vi "Write OCP Enable.vi"(8 "error in":errorcluster, 10 "OCP Enable":bool, 11 "Electronic Load in":refnum<class "Electronic Load.lvclass">) -> (0 "error out":errorcluster, 3 "Electronic Load out":refnum<class "Electronic Load.lvclass">)   [LabVIEW 2019, in "Electronic Load.lvlib" / "Electronic Load.lvclass"]
uses:
  Library/Electronic Load.lvclass
  C:/Users/Public/Documents/Development/builds/Instruments/Instruments.lvlibp/Library/Instruments.lvclass
  Library/Electronic Load.lvclass/Electronic Load.ctl
  builds/Instruments/Instruments.lvlibp/Private/Polymorphic/Special/Event from Boolean.vi
  builds/Instruments/Instruments.lvlibp/Accessors/Command with Logging.vi
  builds/Instruments/Instruments.lvlibp/Library/Instruments.lvclass
  builds/Instruments/Instruments.lvlibp
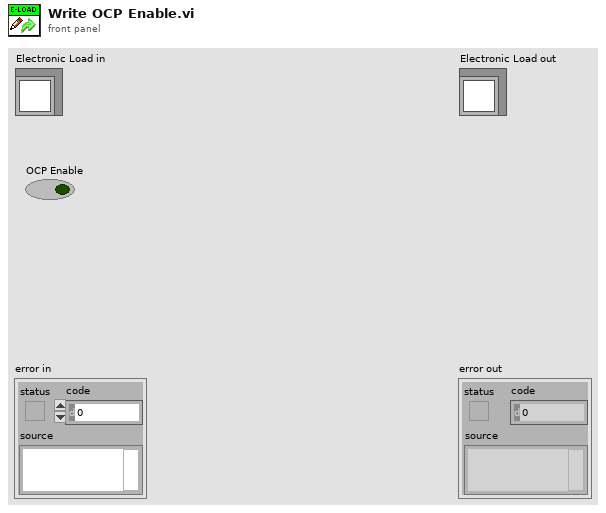
[diagram p1: front panel]
types:
  T1 = typedef "Electronic Load.lvlib/Electronic Load.lvclass/OCP Settings.ctl" = cluster{"OCP_Enabled":bool, "OCP Level":dbl, "OCP Delay":dbl}
  T2 = cluster{"Timestamp":timestamp, "Description":string, "Data":string}
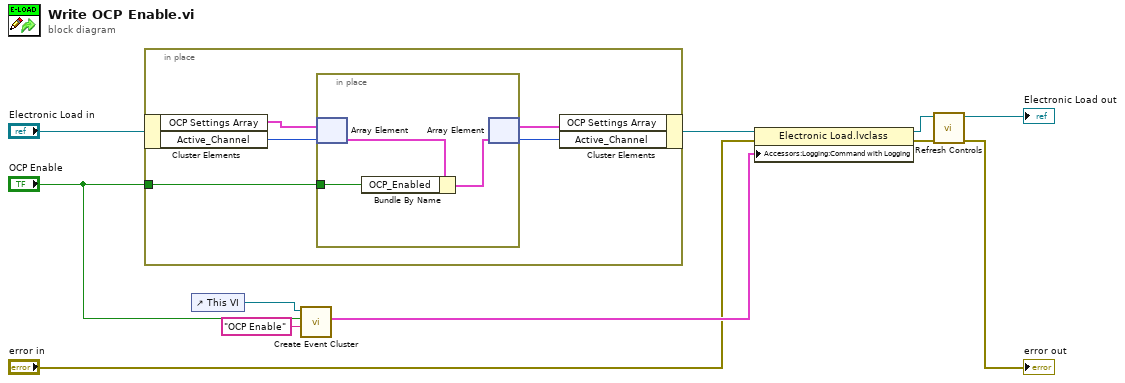
[diagram p0: block diagram]
diagram:
  n1 = in-place {
    in-place-border: "OCP Enable" -> [w12]
    n2 = in-place-cluster #1("Electronic Load in") -> ("OCP Settings Array"=w16:T1[], "Active_Channel"=w15:u32)
    n3 = in-place {
      in-place-border: w12 -> [w17]
      n4 = in-place-array #2(w16, w15) -> (w19:T1)
      n5 = Bundle By Name(cluster=w19, "OCP_Enabled"=w17) -> (w18:T1)
      n6 = in-place-array #2(w18) -> (w14:T1[], w13:i32)
    }
    n7 = in-place-cluster #1("OCP Settings Array"=w14, "Active_Channel"=w13) -> (w9:refnum<class "Electronic Load.lvclass">)
  }
  n8 = control-ref of="This VI"() -> (w10:refnum<vi>)
  n9 = call-poly "Create Event Cluster.vi"("Name"="OCP Enable", "Value"="OCP Enable", "VI Refnum"=w10) -> ("Event Data"=w8:T2)  [unwired: 8 in]
  n10 = property class="Electronic Load.lvclass"(reference=w9, error in="error in", "Accessors:Logging:Command with Logging"=w8) -> (reference out=w3:refnum<class "Electronic Load.lvclass">, error out=w4:errorcluster)
  n11 = call "Refresh Controls.vi"("error in"=w4, "Electronic Load in"=w3) -> ("error out"=→"error out":errorcluster, "Electronic Load out"=→"Electronic Load out":refnum<class "Electronic Load.lvclass">)  [unwired: 8 in]
